vi "Compare File with Master.vi"(8 "error in":errorcluster, 10 "File Index":i32, 11 "Peer Review in":refnum<class "Peer Review.lvclass">) -> (0 "error out":errorcluster, 3 "Peer Review out":refnum<class "Peer Review.lvclass">)   [LabVIEW 2020, in "Peer Review.lvclass"]
uses:
  Peer Review.lvclass
  Peer Review.lvclass/Peer Review.ctl
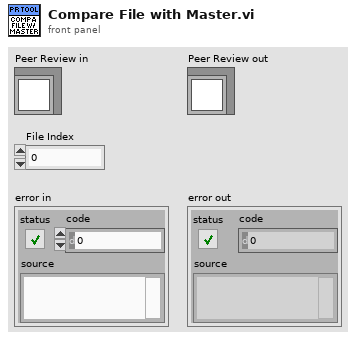
[diagram p1: front panel]
types:
  T1 = typedef "Peer Review.lvclass/File Info.ctl" = cluster{"File ID":i32, "Commit ID":i32, "Reviewed Hash":string, "Relative Path":string, "File Path":path, "File Checksum":string, "State":T2, "FP Changes":i32, "BD Changes":i32, "FP Bounds Error":dbl, "BD Bounds Error":dbl, "Lines Added":i32, "Lines Removed":i32, "Analysis Passes":i32, "Analysis Fails":i32, "Attribute Changes":i32, "Reentrancy State":string, "Cyclomatic Complexity":i32, "Node Count":i32, "Revision Number":u32, "LabVIEW Version":string, "Description":string, "Master Path":path, "Master Checksum":string, "VI Type":T3, "LabVIEW File":bool, "Review Complete":bool, "File Ref":refnum<vi>, "Master Revision":u32}
  T2 = typedef "Peer Review.lvclass/File State.ctl" = enum16{"Interrogation Needed", "Modified", "Deleted", "Added", "Matches Previous", "No Changes", "Moved", "Empty File"}
  T3 = typedef "Peer Review.lvclass/VI Type.ctl" = enum32{"invalid VI type", "Standard VI", "Control VI", "Global VI", "Polymorphic VI", "Configuration VI", "SubSystem", "Facade VI", "Method VI", "Statechart Diagram VI"}
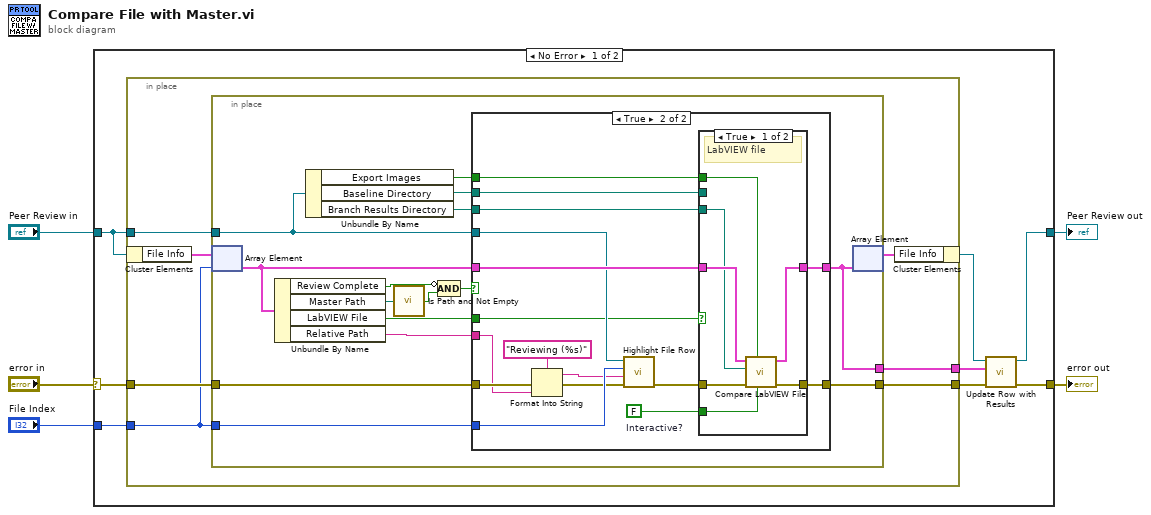
[diagram p0: block diagram]
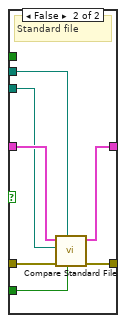
[diagram p3: hidden frame]
diagram:
  n1 = case shown="No Error" "error in" {
    selector: "error in" -> [w11 w69]
    tunnel: [w12 w69] -> w4
    tunnel: "Peer Review in" -> [w8 w68]
    tunnel: "File Index" -> [w13 _]
    tunnel: [w6 w68] -> w1
    frame No Error {
      n2 = in-place {
        in-place-border: w13 -> [w15]
        in-place-border: w11 -> [w20]
        in-place-border: w8 -> [w19]
        in-place-border: [w18] -> w10
        in-place-border: [w17] -> w9
        n3 = in-place-cluster #1(w8) -> ("File Info"=w16:T1[])
        n4 = in-place {
          in-place-border: w15 -> [w33]
          in-place-border: w20 -> [w35]
          in-place-border: w19 -> [w24]
          in-place-border: [w34] -> w18
          in-place-border: [w32] -> w17
          n5 = in-place-array #2(w16, w15) -> (w31:T1)
          n6 = Unbundle By Name(w31) -> ("Review Complete"=w30:bool, "Master Path"=w28:path, "LabVIEW File"=w26:bool, "Relative Path"=w25:string)
          n7 = Unbundle By Name(w24) -> ("Export Images"=w21:bool, "Baseline Directory"=w23:path, "Branch Results Directory"=w22:path)
          n8 = call <vilib>:"Is Path and Not Empty.vi"("path"=w28) -> ("Is Path and Not Empty?"=w27:bool)  [unwired: 4 in]
          n9 = Compound Arithmetic op=AND(invert w30, w27) -> (w29:bool)
          n10 = case shown="True" w29 {
            tunnel: w35 -> [w36 w53]
            tunnel: [w36 w52] -> w34
            tunnel: [w37 w51] -> w32
            tunnel: w24 -> [_ w47]
            tunnel: w33 -> [_ w49]
            tunnel: w31 -> [w37 w48]
            tunnel: w26 -> [_ w42]
            tunnel: w25 -> [_ w41]
            tunnel: w23 -> [_ w40]
            tunnel: w22 -> [_ w39]
            tunnel: w21 -> [_ w38]
            frame False {
              # "Do nothing since this file has already been reviewed or no master to compare against."
            }
            frame True {
              w43 = FALSE  # Interactive?
              n11 = Format Into String(format string="Reviewing (%s)", error in=w53, w41) -> (resulting string=w46:string, error out=w45:errorcluster)  [unwired: 1 in]
              n12 = call "Highlight File Row.vi"("error in"=w45, "Status"=w46, "Current Row"=w49, "Peer Review"=w47) -> ("error out"=w50:errorcluster)  [unwired: 7 in]
              n13 = case shown="True" w42 {
                tunnel: w50 -> [w60 w67]
                tunnel: [w59 w66] -> w52
                tunnel: [w58 w65] -> w51
                tunnel: w43 -> [w55 w63]
                tunnel: w48 -> [w57 w64]
                tunnel: w39 -> [w56 w62]
                tunnel: w40 -> [_ w61]
                tunnel: w38 -> [w54 _]
                frame True {
                  # "LabVIEW file"
                  n14 = call "Compare LabVIEW File.vi"("Interactive?"=w55, "Export Images?"=w54, "error in"=w60, "Results Directory"=w56, "File Info in"=w57) -> ("error out"=w59:errorcluster, "File Info out"=w58:T1)  [unwired: 5 in]
                }
                frame False {
                  # "Standard file"
                  n15 = call "Compare Standard File.vi"("Interactive?"=w63, "Baseline Directory"=w61, "error in"=w67, "Results Directory"=w62, "File Info in"=w64) -> ("error out"=w66:errorcluster, "File Info out"=w65:T1)  [unwired: 5 in]
                }
              }
            }
          }
          n16 = in-place-array #2(w32) -> (w14:T1[])  [unwired: 1 out]
        }
        n17 = in-place-cluster #1("File Info"=w14) -> (w7:refnum<class "Peer Review.lvclass">)
      }
      n18 = call "Update Row with Results.vi"("error in"=w10, "File Info"=w9, "Peer Review in"=w7) -> ("error out"=w12:errorcluster, "Peer Review out"=w6:refnum<class "Peer Review.lvclass">)  [unwired: 7 in]
    }
    frame Error {
    }
  }
  "error out" <- w4
  "Peer Review out" <- w1
